vi "comm close all.vi"(4 "error in (no error)":errorcluster) -> (0 "error out":errorcluster)   [LabVIEW 2013, in "lvserial.lvlib"]
doc: "Closes all serial devices."
uses:
  lvserial.lvlib
  lvserial.dll
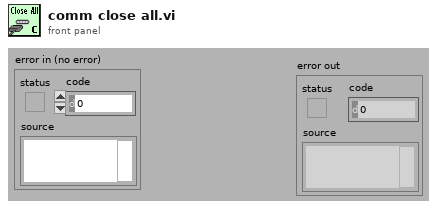
[diagram p1: front panel]
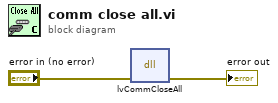
[diagram p0: block diagram]
diagram:
  n1 = dll-call lib="lvserial.dll" fn="lvCommCloseAll"("error in (no error)"="error in (no error)") -> ("error in (no error)"=→"error out":errorcluster)  [unwired: 3 in, 3 out]
